vi "Find Camera Image.vi"() -> ()   [LabVIEW 2016]
uses:
  <vilib>/Rock Robotics/WPI/Camera/WPI_CameraSettings Read MJPG.ctl
  <vilib>/Rock Robotics/WPI/Camera/WPI_CameraImageSize.ctl
panel:
  in  "stop":bool
  out "Image Out":T1(plugin-control)
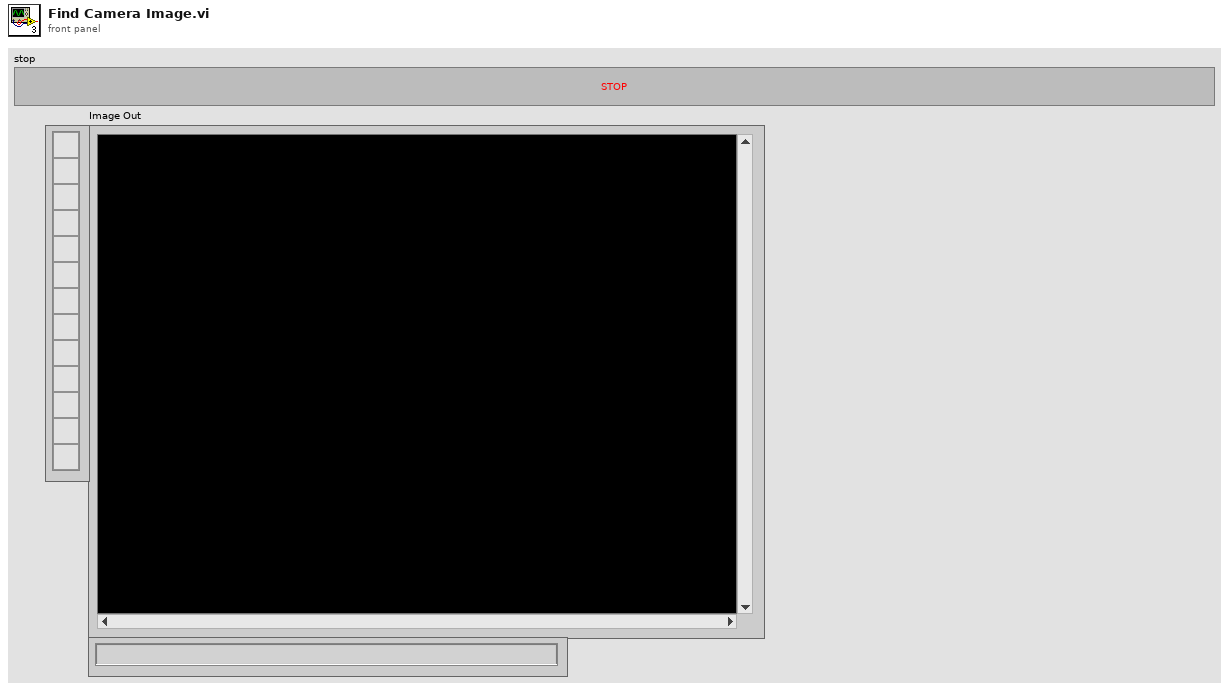
[diagram p1: front panel]
types:
  T1 = typedef "IMAQ Image.ctl" = refnum<image>
  T2 = typedef "Image Type" = u32
  T3 = typedef "WPI_CameraSettings Read MJPG.ctl" = cluster{"fps":i32, "compression":i32, "Image Size":T4, "Config Shown":bool}
  T4 = typedef "WPI_CameraImageSize.ctl" = enum16{"640x480", "320x240", "160x120", "Custom"}
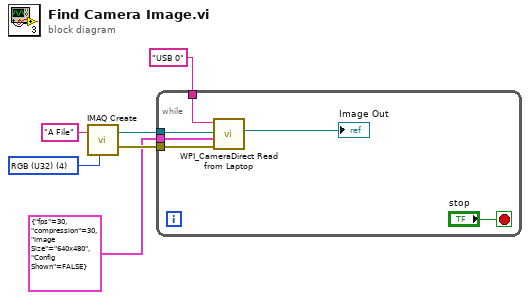
[diagram p0: block diagram]
diagram:
  w1 = T2 4 items=["Grayscale (U8)", "Grayscale (I16)", "Grayscale (SGL)", "Complex (CSG)", "RGB (U32)", "HSL (U32)", "RGB (U64)", "Grayscale (U16)"] ("Image Type")
  n1 = call "IMAQ Create"("Image Name"="A File", "Image Type"=w1) -> ("New Image"=w5:T1, "error out"=w4:errorcluster)  [unwired: 3 in]
  n2 = while {
    tunnel: "USB 0" ("address") -> [w12]
    tunnel: w5 -> [w11]
    tunnel: w4 -> [w10]
    tunnel: T3 {"fps"=30, "compression"=30, "Image Size"=enum."640x480", "Config Shown"=FALSE} ("Camera Settings") -> [w9]
    stop <- "stop" stop-if-true
    n3 = call <vilib>:"WPI_CameraDirect Read from Laptop.vi"("error in"=w10, "Camera Settings"=w9, "Image"=w11, "address"=w12) -> ("Image Out"=→"Image Out":T1)  [unwired: 6 in, 1 out]
  }
